vi "test_get_tool_from_line.vi"() -> ()   [LabVIEW 2017, in "labview-standard-library.lvlib"]
uses:
  labview-standard-library.lvlib
  type-defs/subsystems.ctl
panel:
  out "Array 2":string[](array[string])
  out "Array":T1[](array[typedef])
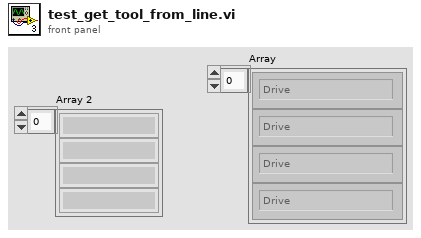
[diagram p1: front panel]
types:
  T1 = typedef "labview-standard-library.lvlib/subsystems.ctl" = enum16{"Drive", "lift", "claw", "invalid"}
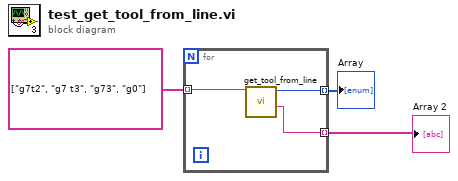
[diagram p0: block diagram]
diagram:
  n1 = for {
    tunnel: string[] ["g7t2", "g7 t3", "g73", "g0"] -> [w6] mode=indexing
    tunnel: [w5] -> w2 mode=indexing
    tunnel: [w4] -> w1 mode=indexing
    n2 = call "get_tool_from_line.vi"("line in"=w6) -> ("line out"=w4:string, "Subsystem out"=w5:T1)  [unwired: 9 in]
  }
  "Array" <- w2
  "Array 2" <- w1
